vi "VK-1701New Coating.vi"(0 "Coating":i32(listbox)) -> (1 "Recipe":string[](array[string]), 2 "Path Array":string[](array[string]))   [LabVIEW 2009]
panel:
  in  "New Coating Tab":enum32{"Page 1"}(tab)
  in  "Add Recipe":bool
  in  "ok":bool
  in  "cancel":bool
  in  "Recipe List Tab":enum32{"Page 1"}(tab)
  in  "Recipe List":i32(listbox)
  in  "Recipe File":path
  in  "Process Name":string
  in  "Move down":bool
  in  "Move up":bool
  in  "delete":bool
  out "error out":errorcluster
  # "Recipe List"
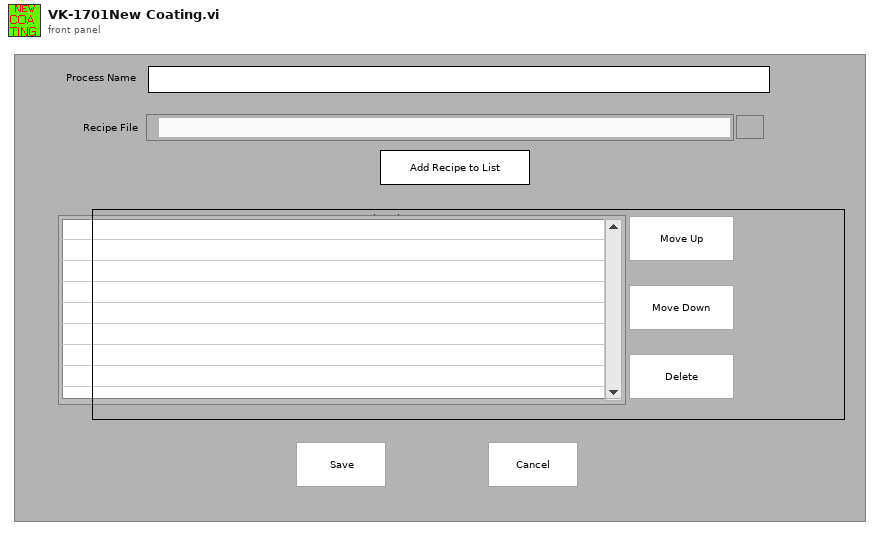
[diagram p1: front panel]
types:
  T1 = enum16{"open", "replace", "create", "open or create", "replace or create", "replace or create with confirmation"}
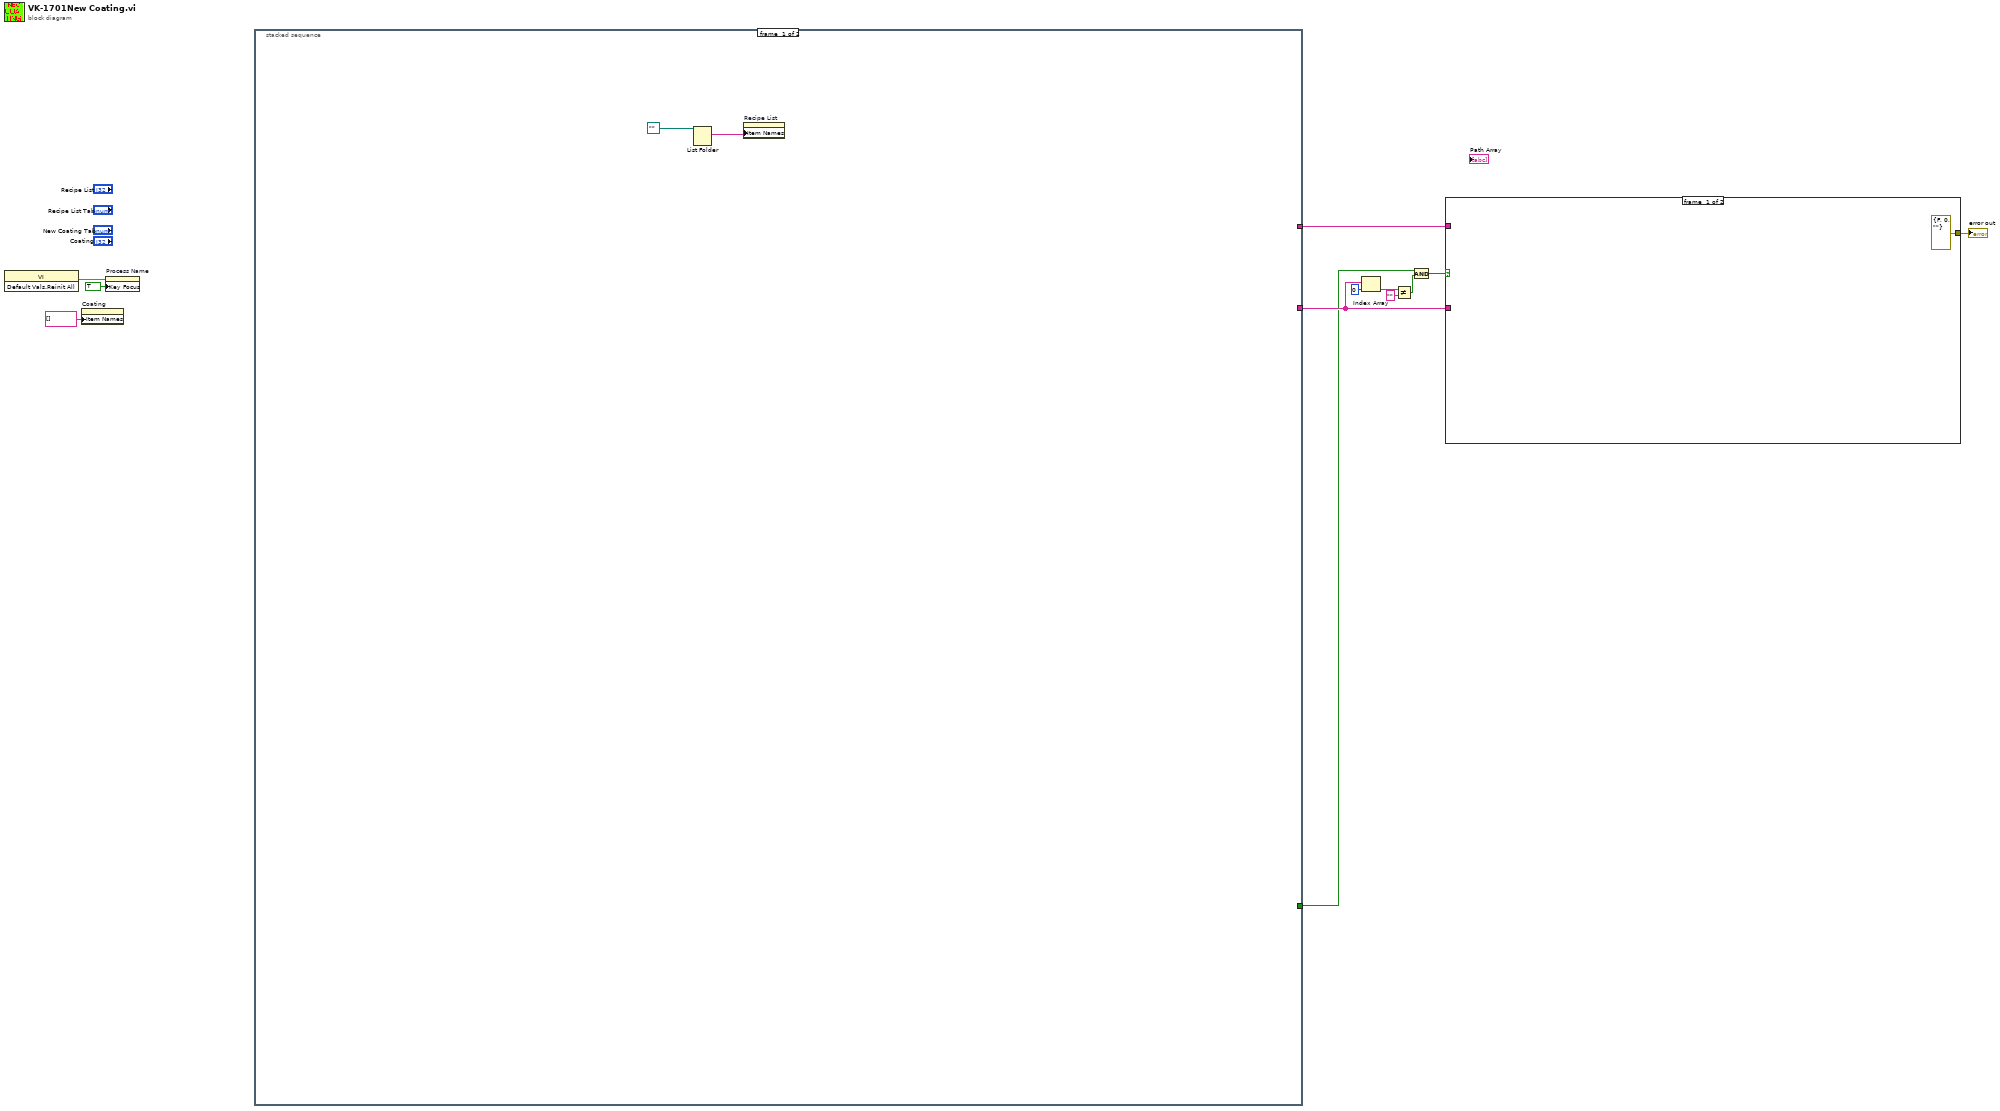
[diagram p0: block diagram]
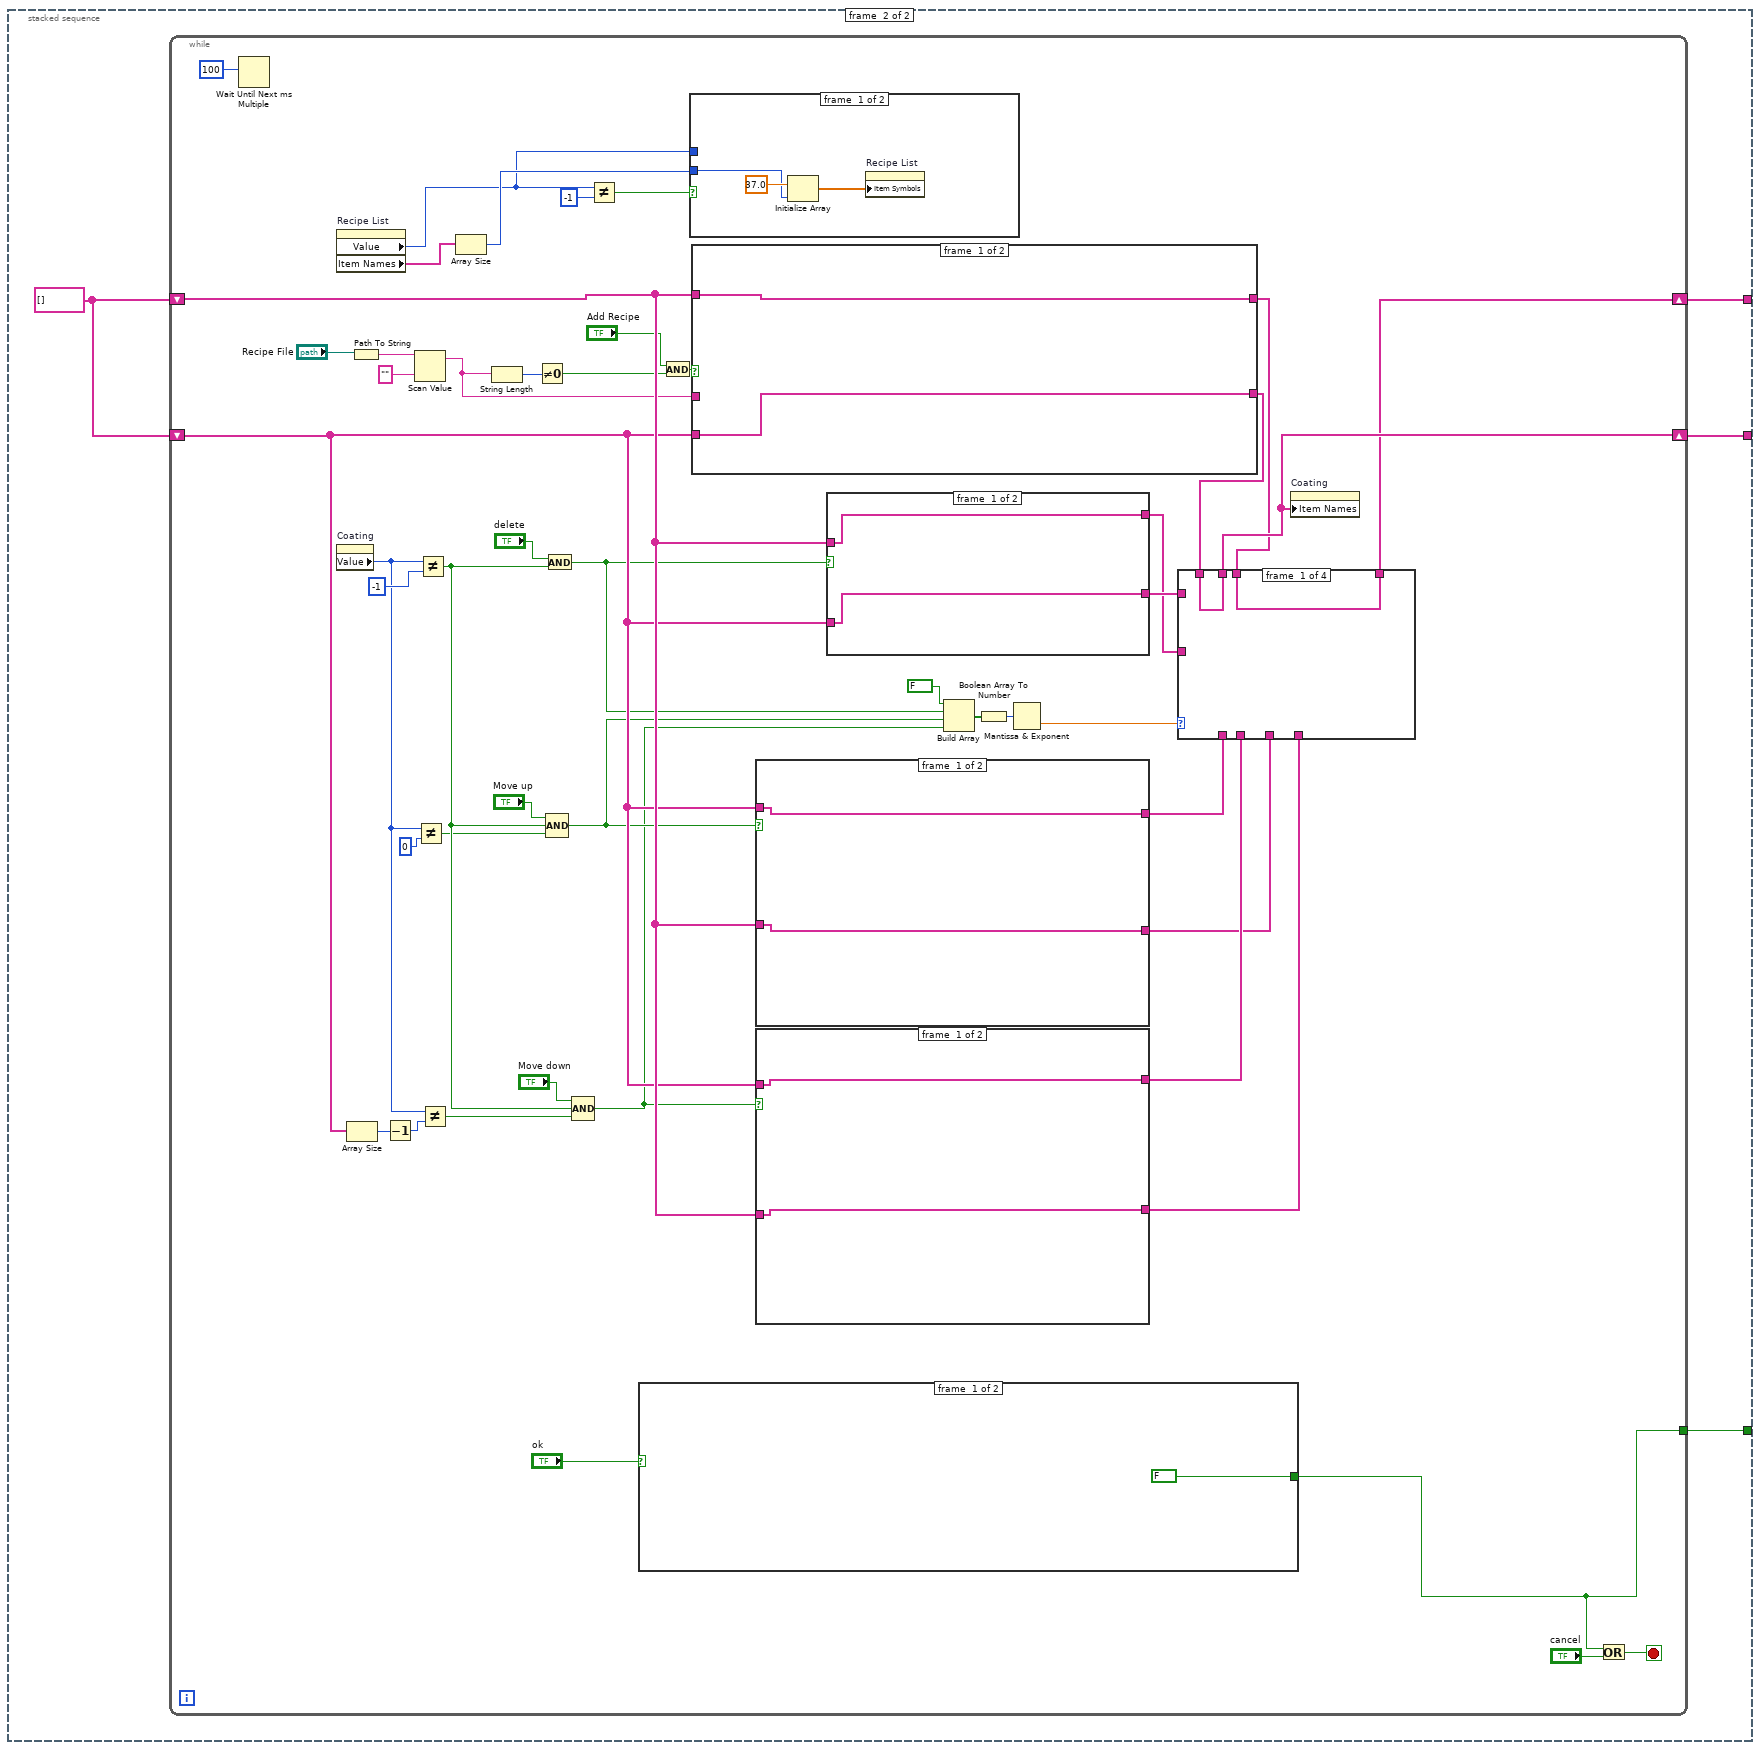
[diagram p2: hidden frame]
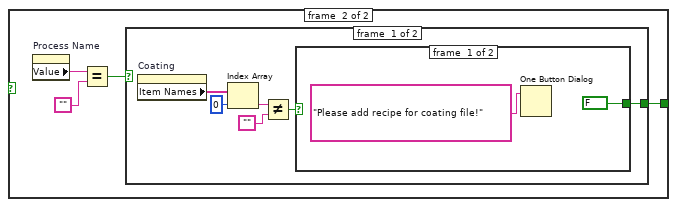
[diagram p3: hidden frame]
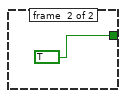
[diagram p4: hidden frame]
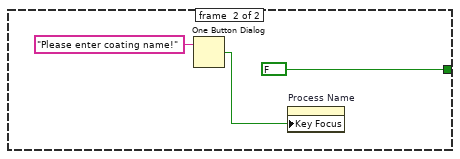
[diagram p5: hidden frame]
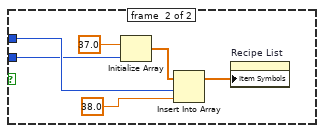
[diagram p6: hidden frame]
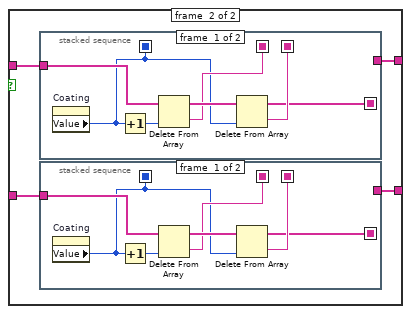
[diagram p10: hidden frame]
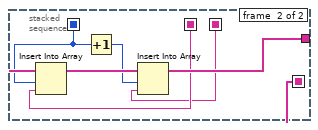
[diagram p11: hidden frame]
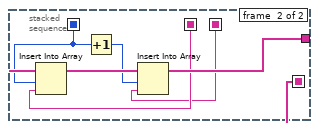
[diagram p12: hidden frame]
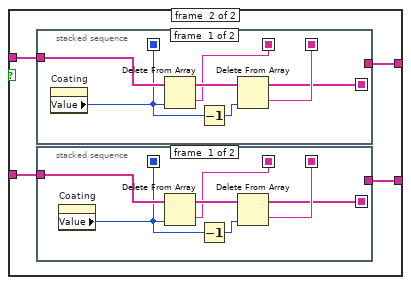
[diagram p13: hidden frame]
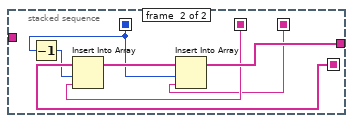
[diagram p14: hidden frame]
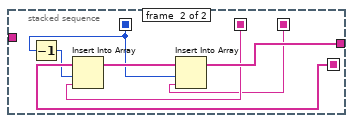
[diagram p15: hidden frame]
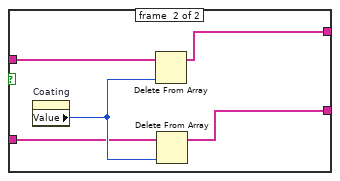
[diagram p16: hidden frame]
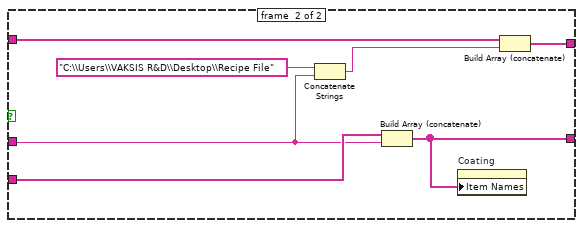
[diagram p17: hidden frame]
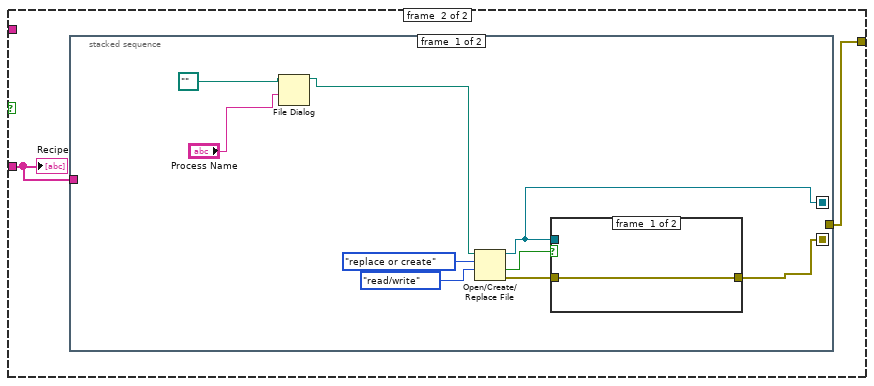
[diagram p18: hidden frame]
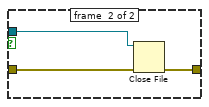
[diagram p19: hidden frame]
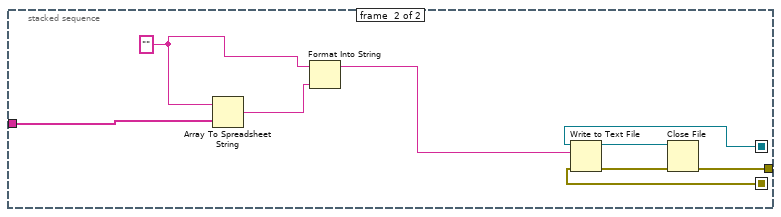
[diagram p20: hidden frame]
diagram:
  n1 = invoke class="VI" method="Default Vals.Reinit All"() -> (error out=w4:errorcluster)  [unwired: 3 in, 2 out]
  n2 = property on="Coating" class="LstBox (strict)"("Item Names"=string[] []) -> ()  [unwired: 2 in, 2 out]
  n3 = property on="Process Name" class="Str"(error in=w4, "Key Focus"=TRUE) -> ()  [unwired: 1 in, 2 out]
  n4 = stacked-sequence {
    tunnel: [_ w17] -> w1
    tunnel: [_ w16] -> w11
    tunnel: [_ w15] -> w2
    frame #0 {
      n5 = List Folder(path=path "") -> (filenames=w13:string[])  [unwired: 3 in, 3 out]
      n6 = property on="Recipe List" class="LstBox (strict)"("Item Names"=w13) -> ()  [unwired: 2 in, 2 out]
    }
    frame #1 {
      w18 = string[] []
      n7 = while {
        shift-right: [w62] -> w17
        shift-left: w18 -> [w63]
        shift-right: [w64] -> w16
        shift-left: w18 -> [w61]
        tunnel: [w60] -> w15
        stop <- w65 stop-if-true
        n8 = Wait Until Next ms Multiple(millisecond multiple=100) -> ()  [unwired: 1 out]
        n9 = property on="Recipe List" class="LstBox (strict)"() -> ("Value"=w27:i32, "Item Names"=w32:string[])  [unwired: 2 in, 2 out]
        n10 = property on="Coating" class="LstBox (strict)"() -> ("Value"=w36:i32)  [unwired: 2 in, 2 out]
        n11 = Array Size(array=w61) -> (size(s)=w35:i32)
        n12 = Path To String(path="Recipe File") -> (string=w23:string)
        n13 = Decrement(x=w35) -> (x-1=w34:i32)
        n14 = Scan Value(string=w23, format string="") -> (output string=w21:string)  [unwired: 1 in, 1 out]
        n15 = Not Equal?(x=w36, y=0) -> (x != y?=w38:bool)
        n16 = Not Equal?(x=w36, y=-1) -> (x != y?=w42:bool)
        n17 = Not Equal?(x=w36, y=w34) -> (x != y?=w37:bool)
        n18 = Array Size(array=w32) -> (size(s)=w30:i32)
        n19 = String Length(string=w21) -> (length=w20:i32)
        n20 = Not Equal To 0?(x=w20) -> (x != 0?=w19:bool)
        n21 = And(x="delete", y=w42) -> (x .and. y?=w45:bool)
        n22 = Compound Arithmetic op=AND("Move up", w42, w38) -> (w43:bool)
        n23 = Compound Arithmetic op=AND("Move down", w42, w37) -> (w40:bool)
        n24 = Not Equal?(x=w27, y=-1) -> (x != y?=w31:bool)
        n25 = case shown="True" "ok" {
          tunnel: [FALSE w68] -> w60
          frame #0 {
          }
          frame #1 {
            n26 = property on="Process Name" class="Str"() -> ("Value"=w70:string)  [unwired: 2 in, 2 out]
            n27 = Equal?(x=w70, y="") -> (x = y?=w69:bool)
            n28 = case shown="False" w69 {
              tunnel: [w72 FALSE] -> w68
              frame #0 {
                n29 = property on="Coating" class="LstBox (strict)"() -> ("Item Names"=w75:string[])  [unwired: 2 in, 2 out]
                n30 = Index Array(array=w75, index=0) -> (element=w77:string)
                n31 = Not Equal?(x=w77, y="") -> (x != y?=w73:bool)
                n32 = case shown="False" w73 {
                  tunnel: [FALSE TRUE] -> w72
                  frame #0 {
                    n33 = One Button Dialog(message="Please add recipe for coating file!") -> ()  [unwired: 1 in, 1 out]
                  }
                  frame #1 {
                  }
                }
              }
              frame #1 {
                n34 = One Button Dialog(message="Please enter coating name!") -> (true=w81:bool)  [unwired: 1 in]
                n35 = property on="Process Name" class="Str"("Key Focus"=w81) -> ()  [unwired: 2 in, 2 out]
              }
            }
          }
        }
        n36 = And(x="Add Recipe", y=w19) -> (x .and. y?=w29:bool)
        n37 = case shown="False" w31 {
          tunnel: w27 -> [_ w89]
          tunnel: w30 -> [w85 w88]
          frame #0 {
            n38 = Initialize Array(37.0 ("element"), w85) -> (w84:dbl[])
            n39 = property on="Recipe List" class="LstBox (strict)"("Item Symbols"=w84) -> ()  [unwired: 2 in, 2 out]
          }
          frame #1 {
            n40 = Initialize Array(37.0 ("element"), w88) -> (w92:dbl[])
            n41 = Insert Into Array(array=w92, index=w89, new element=38.0 ("element")) -> (w87:dbl[])
            n42 = property on="Recipe List" class="LstBox (strict)"("Item Symbols"=w87) -> ()  [unwired: 2 in, 2 out]
          }
        }
        n43 = case shown="True" w29 {
          tunnel: [w177 w182] -> w51
          tunnel: [w176 w181] -> w52
          tunnel: w61 -> [w176 w184]
          tunnel: w63 -> [w177 w183]
          tunnel: w21 -> [_ w179]
          frame #0 {
          }
          frame #1 {
            n44 = Concatenate Strings("C:\\Users\\VAKSIS R&D\\Desktop\\Recipe File" ("string"), w179) -> (w178:string)
            n45 = Build Array (concatenate)(w184, w179) -> (w181:string[])
            n46 = property on="Coating" class="LstBox (strict)"("Item Names"=w181) -> ()  [unwired: 2 in, 2 out]
            n47 = Build Array (concatenate)(w183, w178) -> (w182:string[])
          }
        }
        n48 = case shown="True" w43 {
          tunnel: w61 -> [w136 w140]
          tunnel: [w136 w139] -> w54
          tunnel: w63 -> [w135 w138]
          tunnel: [w135 w137] -> w50
          frame #0 {
          }
          frame #1 {
            n49 = stacked-sequence {
              seq-local: [w158 _] -> [_ w163]
              seq-local: [w157 _] -> [_ w162]
              seq-local: [w156 _] -> [_ w168]
              seq-local: [w155 _] -> [_ w165]
              tunnel: w140 -> [w161 _]
              tunnel: [_ w166] -> w139
              frame #0 {
                n50 = property on="Coating" class="LstBox (strict)"() -> ("Value"=w155:i32)  [unwired: 2 in, 2 out]
                n51 = Delete From Array(array=w161, index=w155) -> (deleted portion=w158:string, array with subset deleted=w160:string[])  [unwired: 1 in]
                n52 = Decrement(x=w155) -> (x-1=w159:i32)
                n53 = Delete From Array(array=w160, index=w159) -> (deleted portion=w157:string, array with subset deleted=w156:string[])  [unwired: 1 in]
              }
              frame #1 {
                n54 = Decrement(x=w165) -> (x-1=w164:i32)
                n55 = Insert Into Array(array=w168, index=w164, new element=w163) -> (w167:string[])
                n56 = Insert Into Array(array=w167, index=w165, new element=w162) -> (w166:string[])
              }
            }
            n57 = stacked-sequence {
              seq-local: [w144 _] -> [_ w149]
              seq-local: [w143 _] -> [_ w148]
              seq-local: [w142 _] -> [_ w154]
              seq-local: [w141 _] -> [_ w151]
              tunnel: w138 -> [w147 _]
              tunnel: [_ w152] -> w137
              frame #0 {
                n58 = property on="Coating" class="LstBox (strict)"() -> ("Value"=w141:i32)  [unwired: 2 in, 2 out]
                n59 = Delete From Array(array=w147, index=w141) -> (deleted portion=w144:string, array with subset deleted=w146:string[])  [unwired: 1 in]
                n60 = Decrement(x=w141) -> (x-1=w145:i32)
                n61 = Delete From Array(array=w146, index=w145) -> (deleted portion=w143:string, array with subset deleted=w142:string[])  [unwired: 1 in]
              }
              frame #1 {
                n62 = Decrement(x=w151) -> (x-1=w150:i32)
                n63 = Insert Into Array(array=w154, index=w150, new element=w149) -> (w153:string[])
                n64 = Insert Into Array(array=w153, index=w151, new element=w148) -> (w152:string[])
              }
            }
          }
        }
        n65 = case shown="True" w40 {
          tunnel: w61 -> [w102 w106]
          tunnel: [w102 w105] -> w53
          tunnel: w63 -> [w101 w104]
          tunnel: [w101 w103] -> w48
          frame #0 {
          }
          frame #1 {
            n66 = stacked-sequence {
              seq-local: [w123 _] -> [_ w131]
              seq-local: [w125 _] -> [_ w130]
              seq-local: [w124 _] -> [_ w134]
              seq-local: [w121 _] -> [_ w128]
              tunnel: w106 -> [w126 _]
              tunnel: [_ w133] -> w105
              frame #0 {
                n67 = property on="Coating" class="LstBox (strict)"() -> ("Value"=w121:i32)  [unwired: 2 in, 2 out]
                n68 = Increment(x=w121) -> (x+1=w122:i32)
                n69 = Delete From Array(array=w126, index=w122) -> (deleted portion=w123:string, array with subset deleted=w127:string[])  [unwired: 1 in]
                n70 = Delete From Array(array=w127, index=w121) -> (deleted portion=w125:string, array with subset deleted=w124:string[])  [unwired: 1 in]
              }
              frame #1 {
                n71 = Insert Into Array(array=w134, index=w128, new element=w131) -> (w132:string[])
                n72 = Increment(x=w128) -> (x+1=w129:i32)
                n73 = Insert Into Array(array=w132, index=w129, new element=w130) -> (w133:string[])
              }
            }
            n74 = stacked-sequence {
              seq-local: [w109 _] -> [_ w117]
              seq-local: [w111 _] -> [_ w116]
              seq-local: [w110 _] -> [_ w120]
              seq-local: [w107 _] -> [_ w114]
              tunnel: w104 -> [w112 _]
              tunnel: [_ w119] -> w103
              frame #0 {
                n75 = property on="Coating" class="LstBox (strict)"() -> ("Value"=w107:i32)  [unwired: 2 in, 2 out]
                n76 = Increment(x=w107) -> (x+1=w108:i32)
                n77 = Delete From Array(array=w112, index=w108) -> (deleted portion=w109:string, array with subset deleted=w113:string[])  [unwired: 1 in]
                n78 = Delete From Array(array=w113, index=w107) -> (deleted portion=w111:string, array with subset deleted=w110:string[])  [unwired: 1 in]
              }
              frame #1 {
                n79 = Insert Into Array(array=w120, index=w114, new element=w117) -> (w118:string[])
                n80 = Increment(x=w114) -> (x+1=w115:i32)
                n81 = Insert Into Array(array=w118, index=w115, new element=w116) -> (w119:string[])
              }
            }
          }
        }
        n82 = case shown="True" w45 {
          tunnel: w63 -> [w169 w175]
          tunnel: w61 -> [w170 w173]
          tunnel: [w170 w172] -> w55
          tunnel: [w169 w171] -> w49
          frame #0 {
          }
          frame #1 {
            n83 = property on="Coating" class="LstBox (strict)"() -> ("Value"=w174:i32)  [unwired: 2 in, 2 out]
            n84 = Delete From Array(array=w175, index=w174) -> (array with subset deleted=w171:string[])  [unwired: 1 in, 1 out]
            n85 = Delete From Array(array=w173, index=w174) -> (array with subset deleted=w172:string[])  [unwired: 1 in, 1 out]
          }
        }
        n86 = Build Array(FALSE, w45, w43, w40) -> (w57:bool[])
        n87 = Boolean Array To Number(Boolean array=w57) -> (number=w58:u32)
        n88 = Mantissa & Exponent(0:w58) -> (2:w56:dbl)  [unwired: 1 out]
        n89 = case shown="0, Default" w56 {
          tunnel: w55 -> [_ w96 _ _]
          tunnel: [w94 w96 w98 w100] -> w64
          tunnel: w54 -> [_ _ w98 _]
          tunnel: w53 -> [_ _ _ w100]
          tunnel: w52 -> [w94 _ _ _]
          tunnel: w51 -> [w93 _ _ _]
          tunnel: [w93 w95 w97 w99] -> w62
          tunnel: w50 -> [_ _ w97 _]
          tunnel: w49 -> [_ w95 _ _]
          tunnel: w48 -> [_ _ _ w99]
          frame #0 {
          }
          frame #1 {
          }
          frame #2 {
          }
          frame #3 {
          }
        }
        n90 = property on="Coating" class="LstBox (strict)"("Item Names"=w64) -> ()  [unwired: 2 in, 2 out]
        n91 = Or(x=w60, y="cancel") -> (x .or. y?=w65:bool)
      }
    }
  }
  n92 = Index Array(array=w11, index=0) -> (element=w9:string)
  n93 = Not Equal?(x=w9, y="") -> (x != y?=w7:bool)
  n94 = Compound Arithmetic op=AND(w2, w7) -> (w6:bool)
  n95 = case shown="True" w6 {
    tunnel: w11 -> [_ w187]
    tunnel: [errorcluster {"status"=FALSE, "code"=0, "source"=""} ("error out") w186] -> w5
    tunnel: w1 -> [_ _]
    frame #0 {
    }
    frame #1 {
      n96 = stacked-sequence {
        seq-local: [w191 _] -> [_ w205]
        seq-local: [w192 _] -> [_ w204]
        tunnel: w187 -> [_ w209]
        tunnel: [_ w203] -> w186
        frame #0 {
          n97 = File Dialog(9:"Process Name", 11:path "" ("base path")) -> (3:w188:path)  [unwired: 2 in, 6 out]
          n98 = Open/Create/Replace File(file path (use dialog)=w188, operation (0:open)=T1."replace or create", access (0:read/write)=enum16{"read/write", "read-only", "write-only"}."read/write") -> (refnum out=w191:refnum<file>, cancelled=w194:bool, error out=w196:errorcluster)  [unwired: 3 in]
          n99 = case shown="True" w194 {
            tunnel: w191 -> [_ w200]
            tunnel: w196 -> [w197 w199]
            tunnel: [w197 w198] -> w192
            frame #0 {
            }
            frame #1 {
              n100 = Close File(refnum=w200, error in=w199) -> (error out=w198:errorcluster)  [unwired: 1 out]
            }
          }
        }
        frame #1 {
          w201 = "" ("format string")
          n101 = Array To Spreadsheet String(array=w209, 3:w201) -> (spreadsheet string=w208:string)  [unwired: 1 in]
          n102 = Format Into String(initial string=w201, w208) -> (resulting string=w206:string)  [unwired: 2 in, 1 out]
          n103 = Write to Text File(file (use dialog)=w205, text=w206, error in=w204) -> (refnum out=w202:refnum<file>, error out=w207:errorcluster)  [unwired: 1 in, 1 out]
          n104 = Close File(refnum=w202, error in=w207) -> (error out=w203:errorcluster)  [unwired: 1 out]
        }
      }
      "Recipe" <- w187
    }
  }
  "error out" <- w5
